vi "CMI ckd2 Get Reference Clock Rate.vi"(8 "error in":errorcluster, 11 "session":T1) -> (0 "error out":errorcluster, 2 "clock rate [Hz]":dbl format="%#_8p", 3 "session out":T1)   [LabVIEW 2020, in "AWG.lvlib"]
doc: "Gets rate of currently selected clock."
uses:
  AWG.lvlib
  CMI ckd2 Session.ctl
  CMI ckd2 Source Mode.ctl
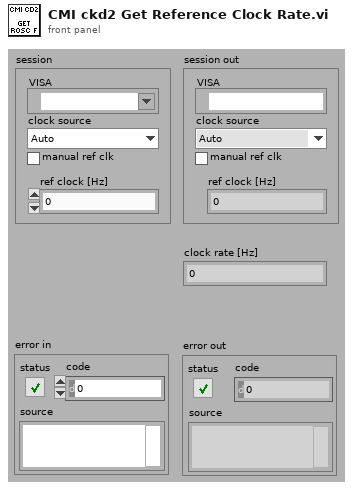
[diagram p1: front panel]
types:
  T1 = typedef "AWG.lvlib/CMI ckd2 Session.ctl" = cluster{"VISA":refnum<visa-resource-name>, "clock source":T2, "manual ref clk":bool, "ref clock [Hz]":dbl}
  T2 = typedef "AWG.lvlib/CMI ckd2 Source Mode.ctl" = enum16{"Auto", "LF clock", "HF clock", "Internal"}
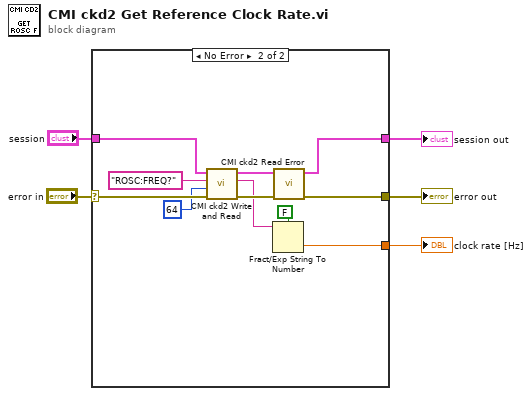
[diagram p0: block diagram]
diagram:
  n1 = case shown="No Error" "error in" {
    selector: "error in" -> [w6 w12]
    tunnel: [w7 w15] -> w3
    tunnel: [w6 w14] -> w5
    tunnel: "session" -> [w7 w18]
    tunnel: [_ w10] -> w1
    frame Error {
    }
    frame No Error {
      n2 = call "CMI ckd2 Write and Read.vi"("error in"=w12, "read byte count (0 - no receive)"=u32 64, "command"="ROSC:FREQ?" ("format string"), "session"=w18) -> ("error out"=w17:errorcluster, "read buffer"=w11:string, "session out"=w16:T1)  [unwired: 5 in]
      n3 = Fract/Exp String To Number(use system decimal point (T)=FALSE, string=w11) -> (number=w10:dbl)  [unwired: 2 in, 1 out]
      n4 = call "CMI ckd2 Read Error.vi"("error in"=w17, "session"=w16) -> ("error out"=w14:errorcluster, "session out"=w15:T1)  [unwired: 7 in, 1 out]
    }
  }
  "error out" <- w5
  "session out" <- w3
  "clock rate [Hz]" <- w1
